vi "Create PV Data.vi"(8 "error in (no error)":errorcluster, 11 "NT Scalar (Numeric) in":refnum<class "NT Scalar (Numeric).lvclass">) -> (0 "error out":errorcluster, 2 "PV Data out":refnum<class "PV Data.lvclass">, 3 "NT Scalar (Numeric) out":refnum<class "NT Scalar (Numeric).lvclass">)   [LabVIEW 2020, in "PV Access.lvlib" / "PV Data.lvlib" / "NT Scalar (Numeric).lvclass"]
uses:
  NT Scalar (Numeric).lvclass
  NT Scalar (Numeric).lvclass/NT Scalar (Numeric).ctl
  PV Data/PV Data.lvclass
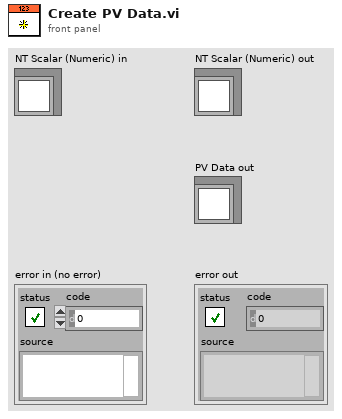
[diagram p1: front panel]
types:
  T1 = typedef "PV Access.lvlib/PV Data.lvlib/Type Code.ctl" = enum8{"Null", "Bool", "BoolA", "Int8", "Int8A", "Int16", "Int16A", "Int32", "Int32A", "Int64", "Int64A", "UInt8", "UInt8A", "UInt16", "UInt16A", "UInt32", "UInt32A", "UInt64", "UInt64A", "Float32", "Float32A", "Float64", "Float64A", "String", "StringA", "Struct", "StructA", "Union", "UnionA", "Any", "AnyA"}
  T2 = typedef "PV Access.lvlib/PV Data.lvlib/Value Fields.ctl" = cluster{"Display":bool, "Control":bool, "Alarm Limits":bool}
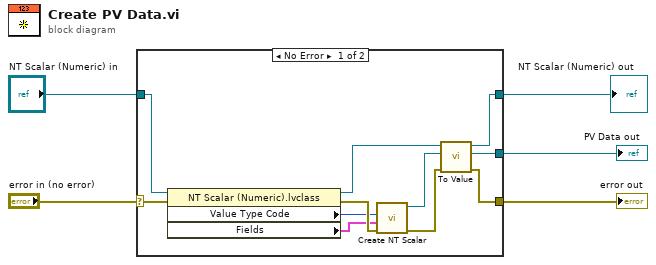
[diagram p0: block diagram]
diagram:
  n1 = case shown="No Error" "error in (no error)" {
    selector: "error in (no error)" -> [w15 w18]
    tunnel: [w9 w18] -> w4
    tunnel: [w6 w17] -> w1
    tunnel: "NT Scalar (Numeric) in" -> [w16 w17]
    tunnel: [w8 _] -> w3
    frame No Error {
      n2 = property class="NT Scalar (Numeric).lvclass"(reference=w16, error in=w15) -> (reference out=w7:refnum<class "NT Scalar (Numeric).lvclass">, error out=w14:errorcluster, "Value Type Code"=w12:T1, "Fields"=w13:T2)
      n3 = call "Create NT Scalar.vi"("error in"=w14, "value fields"=w13, "type code"=w12) -> ("error out"=w10:errorcluster, "PV Data out"=w11:refnum<class "PV Data.lvclass">)  [unwired: 7 in]
      n4 = call-dynamic "To Value.vi"("error in (no error)"=w10, "PV Data in"=w11, "NT Scalar (Numeric) in"=w7) -> ("error out"=w9:errorcluster, "PV Data out"=w8:refnum<class "PV Data.lvclass">, "NT Scalar (Numeric) out"=w6:refnum<class "NT Scalar (Numeric).lvclass">)  [unwired: 6 in]
    }
    frame Error {
    }
  }
  "NT Scalar (Numeric) out" <- w1
  "error out" <- w4
  "PV Data out" <- w3
